vi "setFPGAReference.vi"(10 "FPGAReference":refnum<k20>, 11 "MyHealthAndStatusReadFIFO in":refnum<class "DisplacementDataFIFO.lvclass">) -> (3 "MyHealthAndStatusReadFIFO out":refnum<class "DisplacementDataFIFO.lvclass">)   [LabVIEW 2016, in "DisplacementDataFIFO.lvclass"]
uses:
  DisplacementDataFIFO.lvclass
  DisplacementDataFIFO.lvclass/DisplacementDataFIFO.ctl
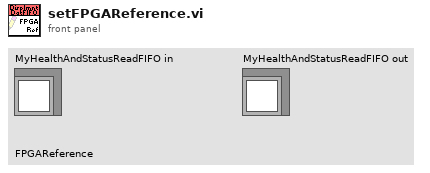
[diagram p1: front panel]
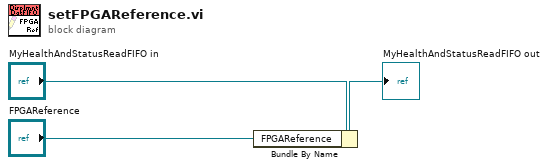
[diagram p0: block diagram]
diagram:
  n1 = Bundle By Name(cluster="MyHealthAndStatusReadFIFO in", "FPGAReference"="FPGAReference") -> (→"MyHealthAndStatusReadFIFO out":refnum<class "DisplacementDataFIFO.lvclass">)
